vi "PH_Sequencer.SCR Start PPMA or Start Middle Fast Devices.vi"(0 "i ref in":refnum<vi>, 5 "error in (no error)":errorcluster) -> (14 "i ref out":refnum<vi>, 19 "error out":errorcluster)   [LabVIEW 2014, in "PH_Sequencer.lvlib"]
doc: "This VI sends a state change request to the Seq SM. If the sequencer is in state \"Start Slow Devices\", and all PPMA PUs are off, \"Start Middle Fast Devices\" is requested; otherwise \"StartPPMA\"."
uses:
  PH_Sequencer.lvlib
  PH_Basics/PH_PP_Common/PH_PP_Common.PUs.ctl
  CS_Core/BaseSM/BaseSM.lvlib
  PH_BeamlineInformation/PH_BeamlineInformation.lvlib
  PH_Basics/PH_PP_Common/PH_PP_Common.lvlib
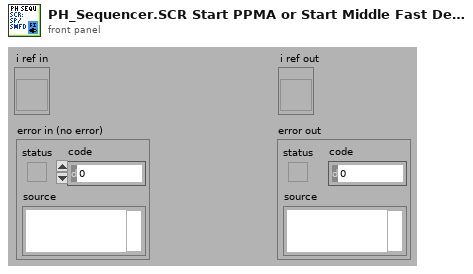
[diagram p1: front panel]
types:
  T1 = typedef "PH_PP_Common.lvlib/PH_PP_Common.PUs.ctl" = enum16{"no Info", "PA-19mm-1", "PA-19mm-2", "PA-45mm-PILC", "PA-45mm-MAIN", "MA-PU-1", "MA-PU-2", "MA-PU-3", "MA-PU-4", "MA-PU-5", "MA-PU-6", "MA-FR", "MA-PILC", "PA-45mm-DP"}
  T2 = typedef "PH_BeamlineInformation.lvlib/PH_BeamlineInformation.i attribute.ctl" = cluster{"BL GUI Elements of Services":cluster{"Service Name":string, "GUI Elements":refnum<vi>[], "Status":i32}[], "Powermeters":T3, "Efficiency":T4, "Heads":T5[]}
  T3 = typedef "PH_BeamlineInformation.lvlib/PH_BeamlineInformation.Powermeter.ctl" = cluster{"ns FE":cluster{"GUI Ref":refnum<vi>, "Value":dbl}, "fs FE":cluster{"GUI Ref":refnum<vi>, "Value":dbl}, "PA":cluster{"GUI Ref":refnum<vi>, "Value":dbl}, "MA":cluster{"GUI Ref":refnum<vi>, "Value":dbl}, "Z6 green":cluster{"GUI Ref":refnum<vi>, "Value":dbl}, "Z6 IR":cluster{"GUI Ref":refnum<vi>, "Value":dbl}, "Z6 COS":cluster{"GUI Ref":refnum<vi>, "Value":dbl}}
  T4 = typedef "PH_BeamlineInformation.lvlib/PH_BeamlineInformation.Efficiency.ctl" = cluster{"PA Gain":cluster{"GUI Ref":refnum<vi>, "Value":dbl}, "MA Gain":cluster{"GUI Ref":refnum<vi>, "Value":dbl}, "Z6 green Conversion":cluster{"GUI Ref":refnum<vi>, "Value":dbl}, "Z6 Comp Losses":cluster{"GUI Ref":refnum<vi>, "Value":dbl}}
  T5 = typedef "PH_BeamlineInformation.lvlib/PH_BeamlineInformation.Head.ctl" = cluster{"PowerUnit":T1, "in use":cluster{"Value":bool, "GUI Ref":refnum<vi>, "linked":bool}, "voltage":cluster{"Value":dbl, "GUI Ref":refnum<vi>, "linked":bool}}
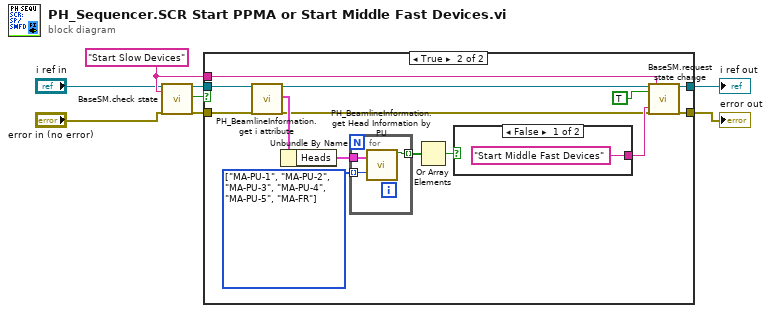
[diagram p0: block diagram]
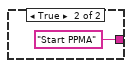
[diagram p3: hidden frame]
diagram:
  w7 = "Start Slow Devices" ("requested state")
  n1 = call "BaseSM.check state.vi"("i ref in"="i ref in", "requestedState"=w7, "error in (no error)"="error in (no error)") -> ("i ref out"=w3:refnum<vi>, "OK"=w1:bool, "error out"=w2:errorcluster)  [unwired: 11 in, 3 out]
  n2 = case shown="True" w1 {
    tunnel: [w9 w22] -> w8
    tunnel: w7 -> [_ w21]
    tunnel: [w10 w19] -> w6
    tunnel: w3 -> [w10 w17]
    tunnel: w2 -> [w9 w16]
    frame False {
    }
    frame True {
      w13 = T1[] [enum."MA-PU-1", enum."MA-PU-2", enum."MA-PU-3", enum."MA-PU-4", enum."MA-PU-5", enum."MA-FR"] items=["no Info", "PA-19mm-1", "PA-19mm-2", "PA-45mm-PILC", "PA-45mm-MAIN", "MA-PU-1", "MA-PU-2", "MA-PU-3", "MA-PU-4", "MA-PU-5", "MA-PU-6", "MA-FR", "MA-PILC", "PA-45mm-DP"]
      n3 = call "PH_BeamlineInformation.get i attribute.vi"("i ref in"=w17, "error in (no error)"=w16) -> ("i ref out"=w15:refnum<vi>, "i attribute"=w20:T2, "error out"=w14:errorcluster)  [unwired: 15 in]
      n4 = Unbundle By Name(w20) -> ("Heads"=w11:T5[])
      n5 = for {
        tunnel: [w27] -> w12 mode=indexing
        tunnel: w13 -> [w26] mode=indexing
        tunnel: w11 -> [w25]
        n6 = call "PH_BeamlineInformation.get Head Information by PU.vi"("Heads"=w25, "Power Unit"=w26) -> ("In Use?"=w27:bool)  [unwired: 12 in, 5 out]
      }
      n7 = Or Array Elements(Boolean array=w12) -> (logical OR=w23:bool)
      n8 = case shown="False" w23 {
        tunnel: ["Start Middle Fast Devices" ("next state") "Start PPMA" ("next state")] -> w24
        frame False {
        }
        frame True {
        }
      }
      n9 = call "BaseSM.request state change.vi"("i ref in"=w15, "change"=TRUE, "error in (no error)"=w14, "allowed current state"=w21, "requested state"=w24) -> ("i ref out"=w19:refnum<vi>, "error out"=w22:errorcluster)  [unwired: 11 in, 2 out]
    }
  }
  "error out" <- w8
  "i ref out" <- w6
